vi "Result_Test.vi"(8 "error in (no error)":errorcluster caption="entrée d'erreur (pas d'erreur)", 11 "Get_Voltage en entrée":refnum<class "Open_ShieldingBox.lvclass">) -> (0 "error out":errorcluster caption="sortie d'erreur", 3 "Get_Voltage en sortie":refnum<class "Open_ShieldingBox.lvclass">)   [LabVIEW 2020, in "Library Test.lvlib" / "Open_ShieldingBox.lvclass"]
uses:
  Open_ShieldingBox.lvclass
  Test/Test_Wtih_Instr/Test_With_Inst.lvclass
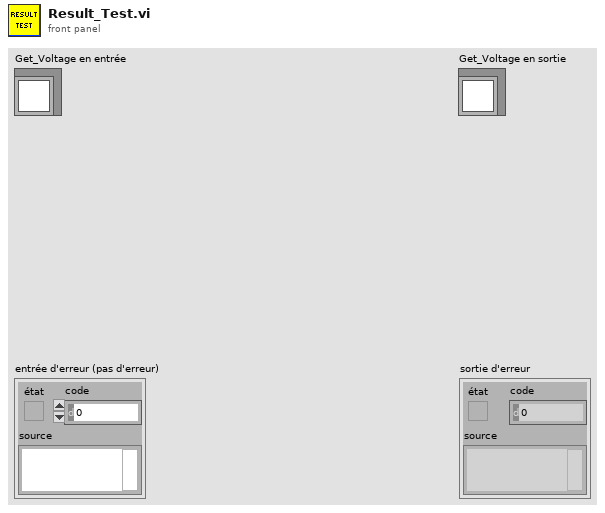
[diagram p1: front panel]
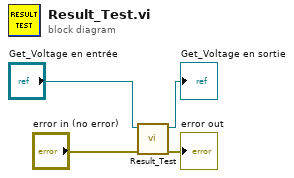
[diagram p0: block diagram]
diagram:
  n1 = call-parent "Result_Test.vi"("error in (no error)"="error in (no error)", "Test_With_Inst en entrée"="Get_Voltage en entrée") -> ("error out"=→"error out":errorcluster, "Test_With_Inst en sortie"=→"Get_Voltage en sortie":refnum<class "Open_ShieldingBox.lvclass">)  [unwired: 8 in]
